vi "Write File.vi"(8 "Error In":errorcluster, 10 "Mux Data Array":T1[](array[typedef]), 11 "Mux File Path":path) -> (0 "Error Out":errorcluster)   [LabVIEW 2013, in "MUX Custom Device.lvlib"]
uses:
  MUX Custom Device.lvlib
  SubVIs/Mux Data.ctl
  SubVIs/Relay Channel Data.ctl
  SubVIs/Relay Data.ctl
  SubVIs/Switch.ctl
  <vilib>/Utility/file.llb/Write To Spreadsheet File (string).vi
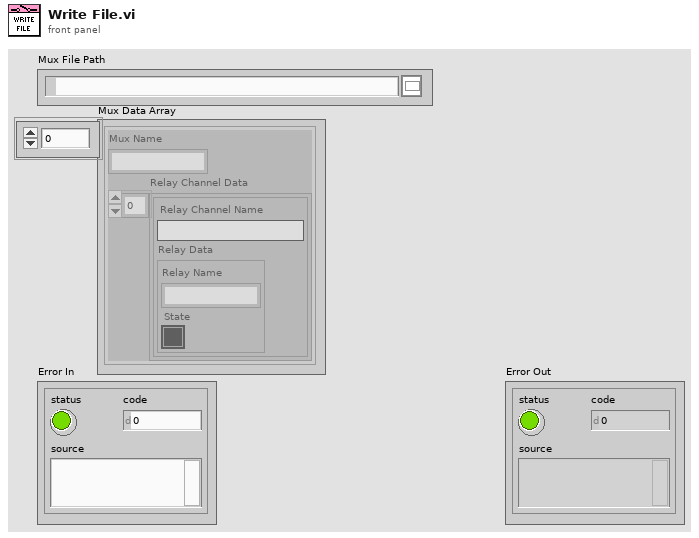
[diagram p1: front panel]
types:
  T1 = typedef "MUX Custom Device.lvlib/Mux Data.ctl" = cluster{"Mux Name":string, "Relay Channel Data":T2[]}
  T2 = typedef "MUX Custom Device.lvlib/Relay Channel Data.ctl" = cluster{"Relay Channel Name":string, "Relay Data":T3}
  T3 = typedef "MUX Custom Device.lvlib/Relay Data.ctl" = cluster{"Relay Name":string, "State":T4}
  T4 = typedef "MUX Custom Device.lvlib/Switch.ctl" = bool
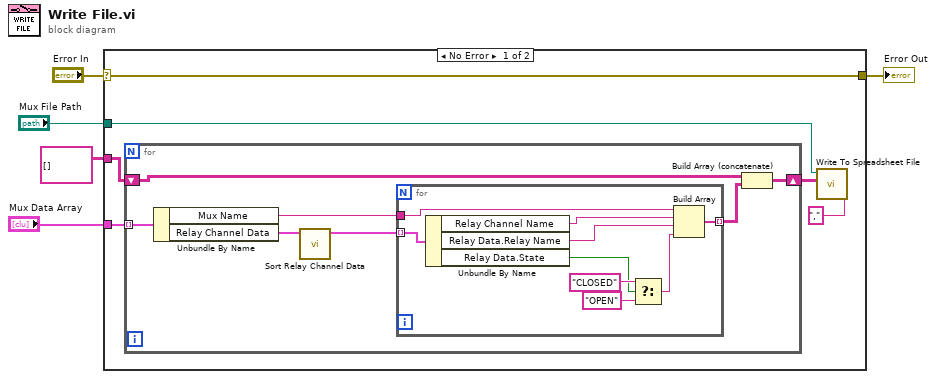
[diagram p0: block diagram]
diagram:
  n1 = case shown="No Error" "Error In" {
    selector: "Error In" -> [w11 w28]
    tunnel: "Mux File Path" -> [w8 _]
    tunnel: [w11 w28] -> w3
    tunnel: "Mux Data Array" -> [w10 _]
    tunnel: string[][] [] -> [w9 _]
    frame No Error {
      n2 = for {
        tunnel: w10 -> [w18] mode=indexing
        shift-right: [w14] -> w7
        shift-left: w9 -> [w16]
        n3 = Unbundle By Name(w18) -> ("Mux Name"=w17:string, "Relay Channel Data"=w13:T2[])
        n4 = call "Sort Relay Channel Data.vi"("Relays"=w13) -> ("Sorted Relays"=w12:T2[])  [unwired: 10 in]
        n5 = for {
          tunnel: w12 -> [w27] mode=indexing
          tunnel: w17 -> [w24]
          tunnel: [w21] -> w15 mode=indexing
          n6 = Unbundle By Name(w27) -> ("Relay Channel Name"=w23:string, "Relay Data.Relay Name"=w20:string, "Relay Data.State"=w19:T4)
          n7 = Select(t="CLOSED" ("true string"), s=w19, f="OPEN" ("false string")) -> (s? t:f=w22:string)
          n8 = Build Array(w24, w23, w20, w22) -> (w21:string[])
        }
        n9 = Build Array (concatenate)(w16, w15) -> (w14:string[][])
      }
      n10 = call-poly <vilib>:"Write To Spreadsheet File.vi"("delimiter (\\t)"="," ("delimiter (\\t)"), "2D data"=w7, "file path (dialog if empty)"=w8) -> ()  [unwired: 5 in, 1 out]
    }
    frame Error {
    }
  }
  "Error Out" <- w3
